vi "Abort Sequence com.vi"(1 "command text in":string[](array[string]), 2 "option":T1) -> (0 "Command text out":string[][](array[string]))   [LabVIEW 2019]
uses:
  Ctl/option.ctl
panel:
  in  "enter":bool
  in  "cancel":bool
  # "Abort Sequence Command"
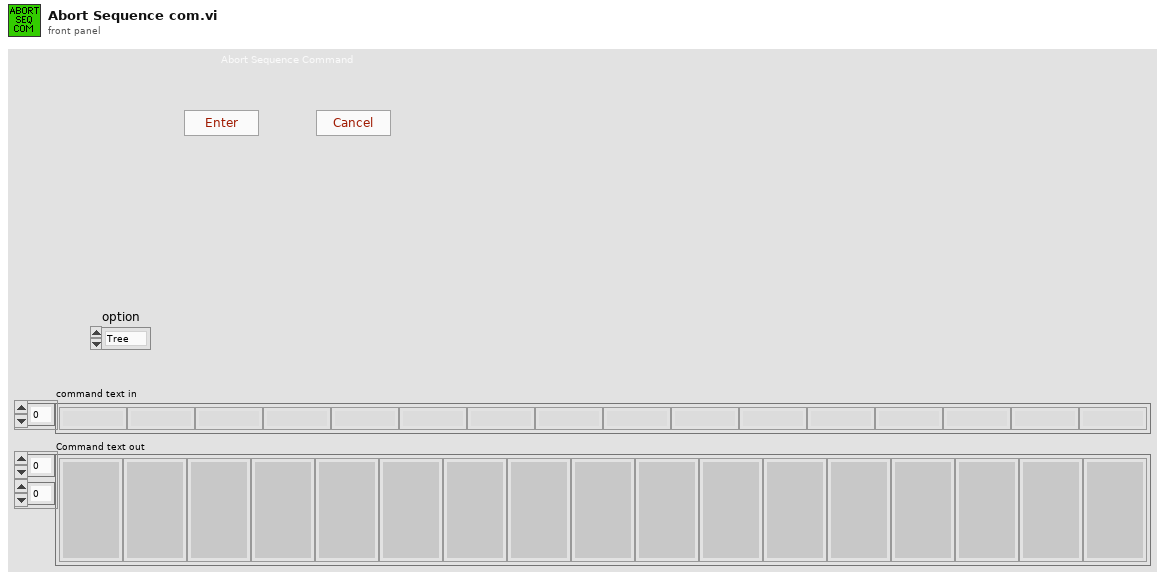
[diagram p1: front panel]
types:
  T1 = typedef "option.ctl" = enum16{"Tree", "List"}
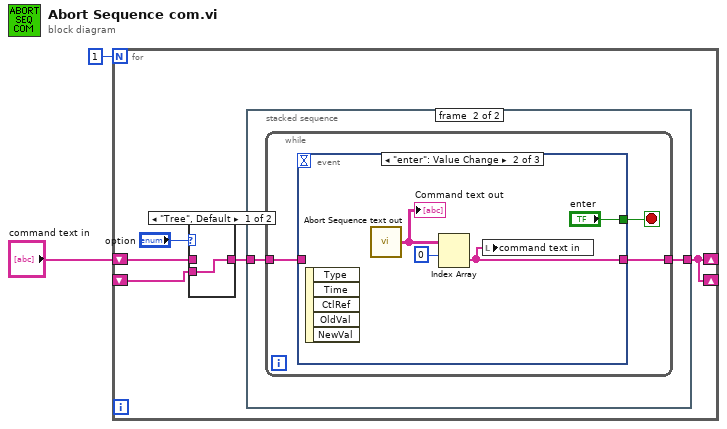
[diagram p0: block diagram]
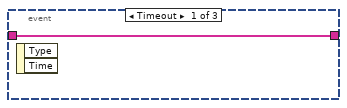
[diagram p4: hidden frame]
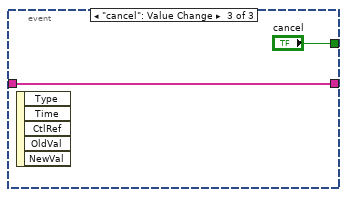
[diagram p5: hidden frame]
diagram:
  n1 = for {
    N: 1 -> [_]
    shift-right: [w3] -> _
    shift-left: "command text in" -> [w6]
    shift-right: [w3] -> _
    shift-left: _ -> [w4]
    n2 = case shown="\"Tree\", Default" "option" {
      tunnel: [w8 w9] -> w5
      tunnel: w4 -> [w8 _]
      tunnel: w6 -> [_ w9]
      frame "Tree", Default {
      }
      frame "List" {
      }
    }
    n3 = stacked-sequence {
      tunnel: [_ w11] -> w3
      tunnel: w5 -> [_ w10]
      frame #0 {
      }
      frame #1 {
        n4 = while {
          tunnel: [w13] -> w11
          tunnel: w10 -> [w12]
          stop <- w14 stop-if-true
          n5 = event shown="[1] \"enter\": Value Change" {
            selector: _ -> [_ _ _]
            dyn-events: _ -> [_ _ _]
            timeout: _ -> [_ _ _]
            tunnel: [_ "enter" "cancel"] -> w14
            tunnel: [w15 w16 w20] -> w13
            tunnel: w12 -> [w15 _ w20]
            event Timeout {
              n6 = event-data() -> ()  [unwired: 1 in, 2 out]
            }
            event "enter": Value Change {
              n7 = event-data() -> ()  [unwired: 1 in, 5 out]
              n8 = call "Abort Sequence text out.vi"() -> ("Command text"=w18:string[][])  [unwired: 4 in]
              "Command text out" <- w18
              n9 = Index Array(array=w18, index (row)=0) -> (element=w16:string[])  [unwired: 1 in]
              n10 = local write "command text in"(w16) -> ()
            }
            event "cancel": Value Change {
              n11 = event-data() -> ()  [unwired: 1 in, 5 out]
            }
          }
        }
      }
    }
  }
